vi "Autonomous Independent.vi"() -> ()   [LabVIEW 2019]
doc: "This VI is called when autonomous begins, and will automatically be terminated when autonomous ends. You can carry out timed or sensor driven robot movement independently without needing to return to the caller."
uses:
  AutoMachine.ctl
  <vilib>/Rock Robotics/WPI/Utilities/WPI_GetSetVariantRefNum.vi
  <vilib>/Rock Robotics/Network Tables/NT Read String.vi
  <vilib>/Rock Robotics/Network Tables/NT Write Numeric Array.vi
  Actuators_n_Sensor_Global.vi
  Axes_n_Buttons_Global.vi
panel:
  in  "Tab Control":T1(tab)=enum."Preparar"
  out "Waveform Chart":cluster{"Distance (m)":dbl, dbl}(graph)={"Distance (m)"=1.5, 1.3199038091281803}
  in  "Precision":dbl
  in  "Distance (m)":dbl=1.5
  in  "Range":cluster{"output high":dbl, "output low":dbl}={"output high"=0.6, "output low"=-0.6} {"output low" format="%.2f"; "output high" format="%.2f"}
  in  "Delay After":i32
  in  "Loop Wait Delay":i32
  out "output cluster":cluster{"Distance (m)":dbl, dbl}={"Distance (m)"=1.5, 1.3199038091281803}
  in  "Gains":T2={"proportional gain (Kc)"=1.0, "integral time (Ti, min)"=0.0, "derivative time (Td, min)"=0.0} {"derivative time (Td, min)" format="%.3f"; "integral time (Ti, min)" format="%.3f"; "proportional gain (Kc)" format="%.3f"}
  in  "Range 2":cluster{"output high":dbl, "output low":dbl}={"output high"=0.75, "output low"=-0.6} {"output low" format="%.2f"; "output high" format="%.2f"}
  in  "Gains 2":T2={"proportional gain (Kc)"=1.0, "integral time (Ti, min)"=0.0, "derivative time (Td, min)"=0.0} {"derivative time (Td, min)" format="%.3f"; "integral time (Ti, min)" format="%.3f"; "proportional gain (Kc)" format="%.3f"}
  in  "Distance (m) 2":dbl=1.45
  in  "Precision 2":dbl=0.3
  in  "Delay After 2":i32
  in  "Loop Wait Delay 2":i32
  out "Waveform Chart 2":cluster{"Distance (m)":dbl, dbl}(graph)={"Distance (m)"=1.45, 1.1995101174675928}
  out "output cluster 2":cluster{"Distance (m)":dbl, dbl}={"Distance (m)"=1.45, 1.1995101174675928}
  in  "Range 3":cluster{"output high":dbl, "output low":dbl}={"output high"=0.8, "output low"=-1.0} {"output low" format="%.2f"; "output high" format="%.2f"}
  in  "Distance (m) 3":dbl=-2.6
  in  "Precision 3":dbl=0.1
  in  "Delay After 3":i32
  in  "Loop Wait Delay 3":i32
  out "Waveform Chart 3":cluster{"Distance (m)":dbl, dbl}(graph)={"Distance (m)"=-2.7, -2.880670114936408}
  out "output cluster 3":cluster{"Distance (m)":dbl, dbl}={"Distance (m)"=-2.7, -2.880670114936408}
  in  "Gains 3":T2={"proportional gain (Kc)"=0.9, "integral time (Ti, min)"=0.0, "derivative time (Td, min)"=0.0} {"derivative time (Td, min)" format="%.3f"; "integral time (Ti, min)" format="%.3f"; "proportional gain (Kc)" format="%.3f"}
  in  "Espera (s)":dbl=2.0
  # "Be sure to right-click and choose Data Operations>>Make Current Value default if you want to save the array values with the VI"
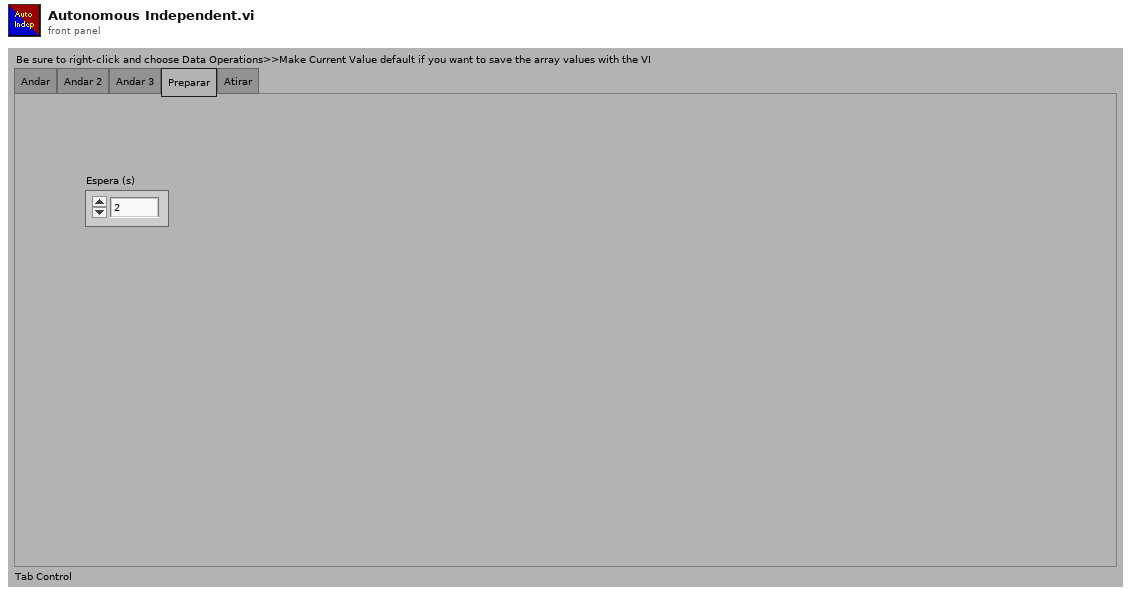
[diagram p1: front panel]
types:
  T1 = enum32{"Andar", "Andar 2", "Andar 3", "Preparar", "Atirar"}
  T2 = cluster{"proportional gain (Kc)":dbl, "integral time (Ti, min)":dbl, "derivative time (Td, min)":dbl}
  T3 = typedef "AutoMachine.ctl" = enum16{"Start", "Andar", "Encoder Reset", "Andar 2", "Encoder Reset 2", "Andar 3", "Ativar LL", "Preparar", "Atirar", "Resetar"}
  T4 = typedef "WPI_JoystickDevRef.ctl" = cluster{"Device":T5}
  T5 = typedef "WPI_JoystickDeviceEnum.ctl" = enum16{"USB 0", "USB 1", "USB 2", "USB 3", "USB 4", "USB 5"}
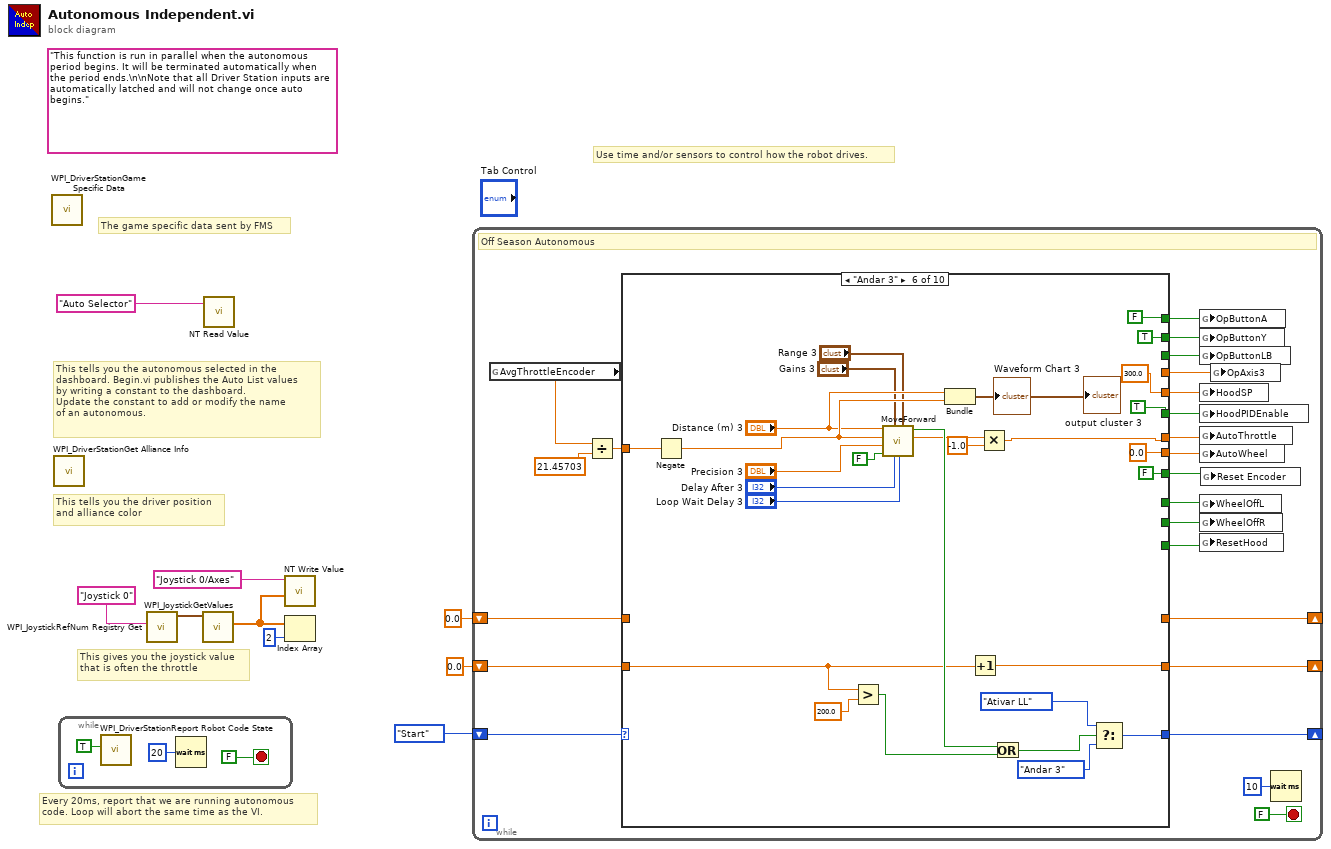
[diagram p0: block diagram]
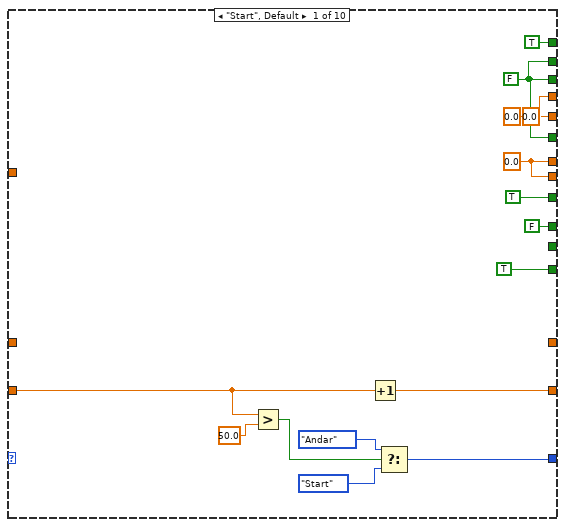
[diagram p2: hidden frame]
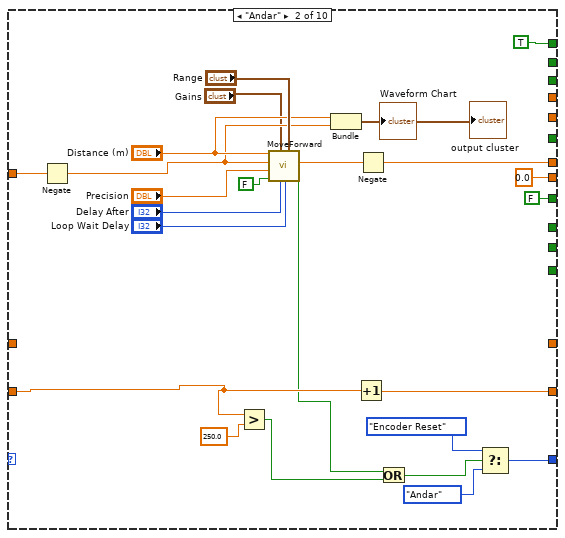
[diagram p3: hidden frame]
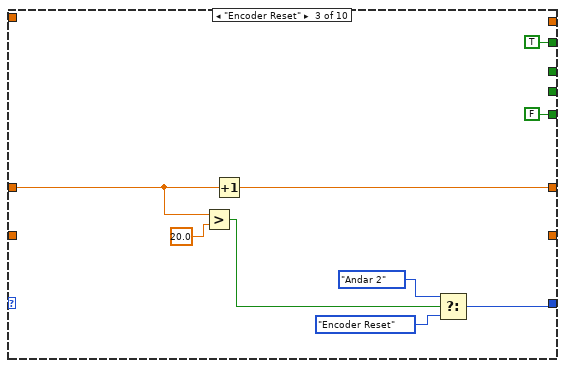
[diagram p4: hidden frame]
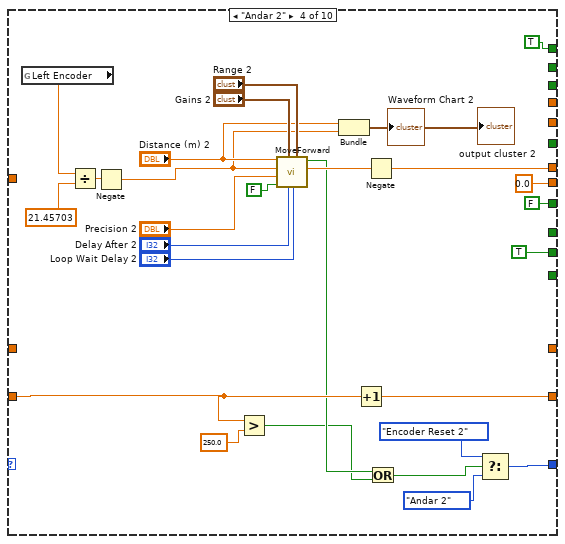
[diagram p5: hidden frame]
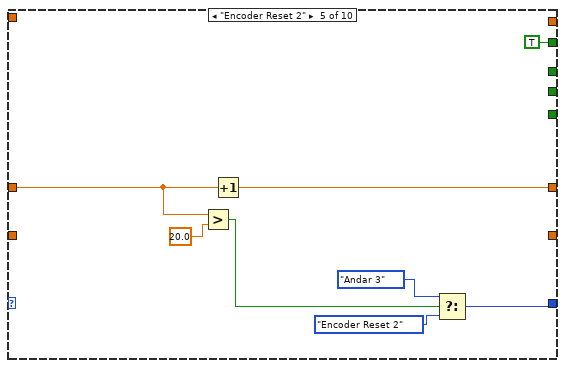
[diagram p6: hidden frame]
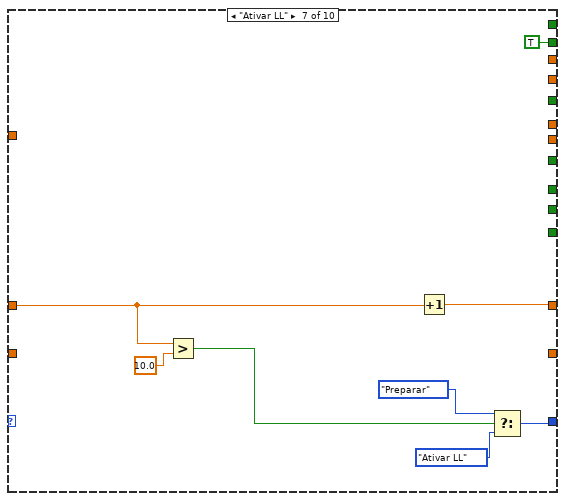
[diagram p7: hidden frame]
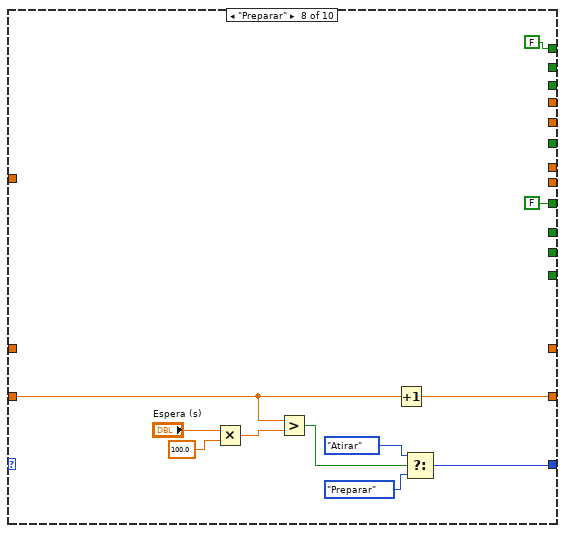
[diagram p8: hidden frame]
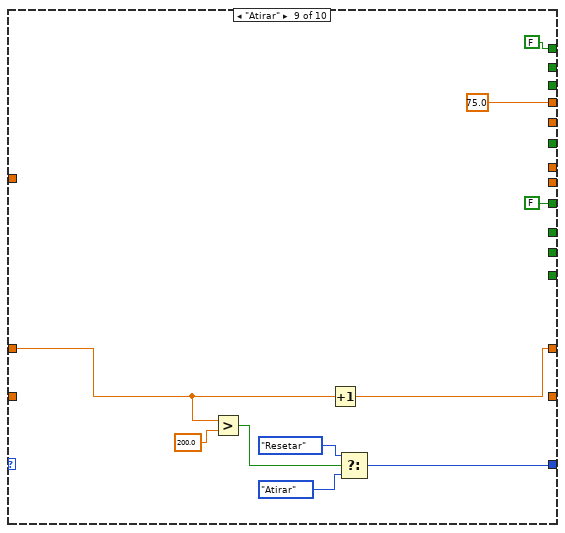
[diagram p9: hidden frame]
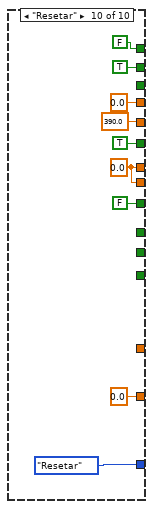
[diagram p10: hidden frame]
diagram:
  (unwired) "This function is run in parallel when the autonomous period begins. It will be terminated automatically when the period ends.\n\nNote that all Driver Station inputs are automatically latched and will not change once auto begins."
  # "The game specific data sent by FMS"
  # "This tells you the autonomous selected in the \ndashboard. Begin.vi publishes the Auto List values\nby writing a constant to the dashboard.\nUpdate the constant to add or modify the name\nof an autonomous."
  # "Every 20ms, report that we are running autonomous\ncode. Loop will abort the same time as the VI."
  # "This gives you the joystick value\nthat is often the throttle"
  # "Use time and/or sensors to control how the robot drives."
  # "This tells you the driver position\nand alliance color"
  n1 = call <vilib>:"WPI_DriverStationGame Specific Data.vi"() -> ()  [unwired: 11 in, 1 out]
  n2 = call <vilib>:"WPI_DriverStationGet Alliance Info.vi"() -> ()  [unwired: 12 out]
  n3 = while {
    stop <- FALSE stop-if-true
    n4 = call <vilib>:"WPI_DriverStationReport Robot Code State.vi"("Autonomous"=TRUE) -> ()  [unwired: 10 in, 1 out]
    n5 = Wait (ms)(milliseconds to wait=u32 20) -> ()  [unwired: 1 out]
  }
  n6 = call <vilib>:"WPI_JoystickRefNum Registry Get.vi"("refnum name"="Joystick 0") -> ("JoystickDevRef"=w8:T4)  [unwired: 1 in, 9 out]
  n7 = call <vilib>:"WPI_JoystickGetValues.vi"("JoystickDevRef"=w8) -> ("Axes"=w5:dbl[])  [unwired: 6 in, 4 out]
  n8 = call-poly <vilib>:"NT Read Value.vi"("Name"="Auto Selector") -> ()  [unwired: 9 in, 2 out]
  n9 = call-poly <vilib>:"NT Write Value.vi"("Numeric Array"=w5, "Name"="Joystick 0/Axes") -> ()  [unwired: 9 in, 1 out]
  n10 = Index Array(array=w5, index=2) -> ()  [unwired: 1 out]
  n11 = while {
    shift-right: [w14] -> _
    shift-left: AutoMachine."Start" -> [w33]
    shift-right: [w27] -> _
    shift-left: 0.0 -> [w26]
    shift-right: [w15] -> _
    shift-left: 0.0 -> [w16]
    stop <- FALSE stop-if-true
    # "Off Season Autonomous"
    n12 = global read "Actuators_n_Sensor_Global.vi" "AvgThrottleEncoder"() -> (w23:dbl)
    n13 = Divide(x=w23, y=21.45703) -> (x/y=w22:dbl)
    n14 = case shown="\"Andar 3\"" w33 {
      tunnel: [w40 w51 w76 w84 w112 w126 w150 w159 w172 AutoMachine."Resetar"] -> w14
      tunnel: [w50 w62 _ w95 _ w122 _ _ _ w182] -> w32
      tunnel: [w50 0.0 _ 0.0 _ 0.0 _ _ _ w182] -> w31
      tunnel: [w37 _ _ _ _ _ TRUE _ _ _] -> w30
      tunnel: [w37 _ _ _ _ TRUE _ _ _ TRUE] -> w29
      tunnel: [0.0 ("Output") _ _ _ _ 300.0 ("Output") _ _ _ 390.0 ("Output")] -> w28
      tunnel: [w46 w59 _ w96 _ w131 _ w155 _ 0.0] -> w27
      tunnel: w26 -> [w45 w58 _ w97 _ w130 _ w156 _ _]
      tunnel: [w37 _ _ _ _ TRUE _ _ _ TRUE] -> w25
      tunnel: w22 -> [_ w65 _ _ _ w132 _ _ _ _]
      tunnel: [0.0 ("Output") _ _ _ _ _ _ _ 75.0 ("Output") 0.0 ("Output")] -> w21
      tunnel: [TRUE ("OpButtonY") TRUE ("OpButtonY") _ TRUE ("OpButtonY") _ FALSE ("OpButtonY") _ FALSE ("OpButtonY") FALSE ("OpButtonY") FALSE ("OpButtonY")] -> w20
      tunnel: [TRUE ("OpButtonA") FALSE ("OpButtonA") TRUE ("OpButtonA") FALSE ("OpButtonA") TRUE ("OpButtonA") FALSE ("OpButtonA") _ FALSE ("OpButtonA") FALSE ("OpButtonA") FALSE ("OpButtonA")] -> w19
      tunnel: [FALSE ("OpButtonA") _ _ _ _ _ _ _ _ _] -> w18
      tunnel: [_ _ _ TRUE ("OpButtonA") _ _ _ _ _ _] -> w17
      tunnel: w16 -> [_ _ w81 _ w114 _ w148 _ w167 _]
      tunnel: [_ _ w80 _ w113 _ w147 _ w166 _] -> w15
      tunnel: [TRUE ("OpButtonA") _ FALSE ("OpButtonA") _ _ _ _ _ _ _] -> w13
      frame "Start", Default {
        w50 = 0.0 ("Output")
        w37 = FALSE
        n15 = Greater?(x=w45, y=50.0) -> (0:w49:bool)
        n16 = Increment(x=w45) -> (x+1=w46:dbl)
        n17 = Select(t=AutoMachine."Andar", s=w49, f=AutoMachine."Start") -> (s? t:f=w40:T3)
      }
      frame "Andar" {
        n18 = Negate(x=w65) -> (-x=w61:dbl)
        n19 = Greater?(x=w58, y=250.0) -> (0:w54:bool)
        n20 = call "MoveForward.vi"("Loop Wait Delay"="Loop Wait Delay", "Range"="Range", "Delay After"="Delay After", "Gains"="Gains", "Reset"=FALSE, "Precision"="Precision", "Encoder Count"=w61, "Distance"="Distance (m)") -> ("Output"=w72:dbl, "Finished?"=w55:bool)  [unwired: 2 in]
        n21 = Bundle("Distance (m)"="Distance (m)", w61) -> (→"Waveform Chart" →"output cluster":cluster{"Distance (m)":dbl, dbl})  [unwired: 1 in]
        n22 = Increment(x=w58) -> (x+1=w59:dbl)
        n23 = Negate(x=w72) -> (-x=w62:dbl)
        n24 = Or(x=w55, y=w54) -> (x .or. y?=w53:bool)
        n25 = Select(t=AutoMachine."Encoder Reset", s=w53, f=AutoMachine."Andar") -> (s? t:f=w51:T3)
      }
      frame "Encoder Reset" {
        n26 = Greater?(x=w81, y=20.0) -> (0:w79:bool)
        n27 = Increment(x=w81) -> (x+1=w80:dbl)
        n28 = Select(t=AutoMachine."Andar 2", s=w79, f=AutoMachine."Encoder Reset") -> (s? t:f=w76:T3)
      }
      frame "Andar 2" {
        n29 = global read "Actuators_n_Sensor_Global.vi" "Left Encoder"() -> (w90:dbl)
        n30 = Divide(x=w90, y=21.45703) -> (x/y=w88:dbl)
        n31 = Negate(x=w88) -> (-x=w99:dbl)
        n32 = Greater?(x=w97, y=250.0) -> (0:w86:bool)
        n33 = call "MoveForward.vi"("Loop Wait Delay"="Loop Wait Delay 2", "Range"="Range 2", "Delay After"="Delay After 2", "Gains"="Gains 2", "Reset"=FALSE, "Precision"="Precision 2", "Encoder Count"=w99, "Distance"="Distance (m) 2") -> ("Output"=w108:dbl, "Finished?"=w87:bool)  [unwired: 2 in]
        n34 = Bundle("Distance (m) 2"="Distance (m) 2", w99) -> (→"Waveform Chart 2" →"output cluster 2":cluster{"Distance (m) 2":dbl, dbl})  [unwired: 1 in]
        n35 = Increment(x=w97) -> (x+1=w96:dbl)
        n36 = Negate(x=w108) -> (-x=w95:dbl)
        n37 = Or(x=w87, y=w86) -> (x .or. y?=w85:bool)
        n38 = Select(t=AutoMachine."Encoder Reset 2", s=w85, f=AutoMachine."Andar 2") -> (s? t:f=w84:T3)
      }
      frame "Encoder Reset 2" {
        n39 = Greater?(x=w114, y=20.0) -> (0:w117:bool)
        n40 = Increment(x=w114) -> (x+1=w113:dbl)
        n41 = Select(t=AutoMachine."Andar 3", s=w117, f=AutoMachine."Encoder Reset 2") -> (s? t:f=w112:T3)
      }
      frame "Andar 3" {
        n42 = Negate(x=w132) -> (-x=w143:dbl)
        n43 = Greater?(x=w130, y=200.0) -> (0:w145:bool)
        n44 = call "MoveForward.vi"("Loop Wait Delay"="Loop Wait Delay 3", "Range"="Range 3", "Delay After"="Delay After 3", "Gains"="Gains 3", "Reset"=FALSE, "Precision"="Precision 3", "Encoder Count"=w143, "Distance"="Distance (m) 3") -> ("Output"=w124:dbl, "Finished?"=w144:bool)  [unwired: 2 in]
        n45 = Bundle("Distance (m) 3"="Distance (m) 3", w143) -> (→"Waveform Chart 3" →"output cluster 3":cluster{"Distance (m) 3":dbl, dbl})  [unwired: 1 in]
        n46 = Increment(x=w130) -> (x+1=w131:dbl)
        n47 = Multiply(x=w124, y=-1.0) -> (x*y=w122:dbl)
        n48 = Or(x=w144, y=w145) -> (x .or. y?=w146:bool)
        n49 = Select(t=AutoMachine."Ativar LL", s=w146, f=AutoMachine."Andar 3") -> (s? t:f=w126:T3)
      }
      frame "Ativar LL" {
        n50 = Greater?(x=w148, y=10.0) -> (0:w151:bool)
        n51 = Increment(x=w148) -> (x+1=w147:dbl)
        n52 = Select(t=AutoMachine."Preparar", s=w151, f=AutoMachine."Ativar LL") -> (s? t:f=w150:T3)
      }
      frame "Preparar" {
        n53 = Multiply(x="Espera (s)", y=100.0) -> (x*y=w160:dbl)
        n54 = Greater?(x=w156, y=w160) -> (0:w164:bool)
        n55 = Increment(x=w156) -> (x+1=w155:dbl)
        n56 = Select(t=AutoMachine."Atirar", s=w164, f=AutoMachine."Preparar") -> (s? t:f=w159:T3)
      }
      frame "Atirar" {
        n57 = Greater?(x=w167, y=200.0) -> (0:w175:bool)
        n58 = Increment(x=w167) -> (x+1=w166:dbl)
        n59 = Select(t=AutoMachine."Resetar", s=w175, f=AutoMachine."Atirar") -> (s? t:f=w172:T3)
      }
      frame "Resetar" {
        w182 = 0.0 ("Output")
      }
    }
    n60 = global write "Axes_n_Buttons_Global.vi" "OpButtonA"(w20) -> ()
    n61 = global write "Axes_n_Buttons_Global.vi" "OpButtonY"(w25) -> ()
    n62 = global write "Axes_n_Buttons_Global.vi" "OpButtonLB"(w30) -> ()
    n63 = global write "Actuators_n_Sensor_Global.vi" "HoodSP"(w28) -> ()
    n64 = global write "Actuators_n_Sensor_Global.vi" "HoodPIDEnable"(w29) -> ()
    n65 = global write "Axes_n_Buttons_Global.vi" "AutoThrottle"(w32) -> ()
    n66 = global write "Axes_n_Buttons_Global.vi" "AutoWheel"(w31) -> ()
    n67 = global write "Axes_n_Buttons_Global.vi" "WheelOffL"(w18) -> ()
    n68 = global write "Axes_n_Buttons_Global.vi" "WheelOffR"(w17) -> ()
    n69 = global write "Actuators_n_Sensor_Global.vi" "ResetHood"(w13) -> ()
    n70 = global write "Actuators_n_Sensor_Global.vi" "Reset Encoder"(w19) -> ()
    n71 = global write "Axes_n_Buttons_Global.vi" "OpAxis3"(w21) -> ()
    n72 = Wait (ms)(milliseconds to wait=u32 10) -> ()  [unwired: 1 out]
  }
